vi "Generate config String.vi"() -> (2 "JSON string":string="{\"client\":\"wqe\",\"broker\":{\"address\":\"192.168.20.1\",\"port\":1883,\"connTimeout\":2000,\"writeTimeout\":2000,\"readTimeout\":2000,\"subTimeout\":3000},\"connFlags\":{\"reserved\":false,\"clean session\":true,\"will flag\":false,\"willQOS\":\"At least once\",\"will retain\":false,\"password\":true,\"user name\":true},\"User Info\":{\"User Name\":\"homeassistant\",\"Password\":\"SaDyBa13E\"}}")   [LabVIEW 2015, in "MQTTclient.lvclass"]
uses:
  MQTTclient.lvclass
  config.ctl
panel:
  in  "Config":T1={"client"="", "broker"={"address"="", "port"=1883, "connTimeout"=2000, "writeTimeout"=2000, "readTimeout"=0, "subTimeout"=3000}, "connFlags"={"reserved"=FALSE, "clean session"=FALSE, "will flag"=FALSE, "willQOS"="At least once", "will retain"=FALSE, "password"=TRUE, "user name"=TRUE}, "User Info"={"User Name"="", "Password"=""}}
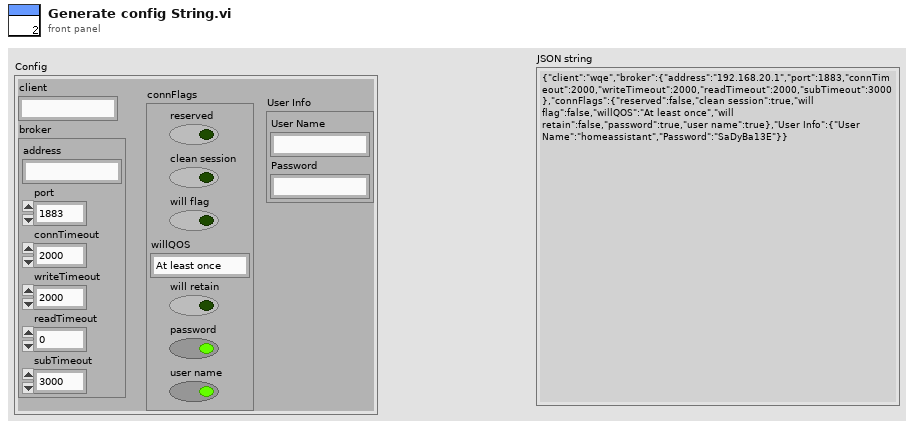
[diagram p1: front panel]
types:
  T1 = typedef "MQTTclient.lvclass/config.ctl" = cluster{"client":string, "broker":cluster{"address":string, "port":u16, "connTimeout":i32, "writeTimeout":i32, "readTimeout":i32, "subTimeout":i32}, "connFlags":cluster{"reserved":bool, "clean session":bool, "will flag":bool, "willQOS":string, "will retain":bool, "password":bool, "user name":bool}, "User Info":cluster{"User Name":string, "Password":string}}
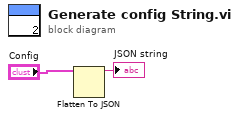
[diagram p0: block diagram]
diagram:
  n1 = Flatten To JSON(anything="Config") -> (JSON string=→"JSON string":string)  [unwired: 2 in, 1 out]
